vi "read_raster_image.vi"(8 "error in (no error)":errorcluster, 11 "scan_2d_hdf5_log in":refnum<class "scan_2d_hdf5_log.lvclass">) -> (0 "error out":errorcluster, 2 "raster_image":dbl[][](array[numeric]), 3 "scan_2d_hdf5_log out":refnum<class "scan_2d_hdf5_log.lvclass">)   [LabVIEW 2015, in "scan_2d_hdf5_log.lvclass"]
uses:
  scan_2d_hdf5_log.lvclass
  scan_2d_hdf5_log.lvclass/scan_2d_hdf5_log.ctl
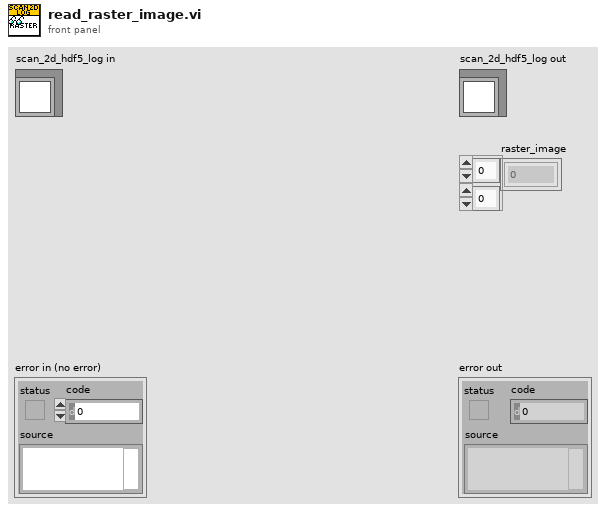
[diagram p1: front panel]
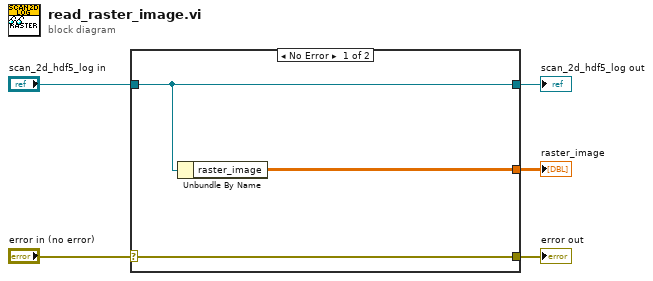
[diagram p0: block diagram]
diagram:
  n1 = case shown="No Error" "error in (no error)" {
    selector: "error in (no error)" -> [w8 w9]
    tunnel: [w8 w9] -> w4
    tunnel: [w7 w10] -> w2
    tunnel: "scan_2d_hdf5_log in" -> [w7 w10]
    tunnel: [w6 _] -> w1
    frame No Error {
      n2 = Unbundle By Name(w7) -> ("raster_image"=w6:dbl[][])
    }
    frame Error {
    }
  }
  "error out" <- w4
  "scan_2d_hdf5_log out" <- w2
  "raster_image" <- w1
